vi "LoadShotSetting.vi"(10 "Shot Number":i32, 11 "Experiment State in":T17={"error"={"status"=FALSE, "code"=0, "source"=""}, "Digitizer DAQmx Tasks"={"TaskArray"=[]}, "DAQ Settings"={"Channel Settings"=[], "Card Settings"=[]}, "Synchronization Settings"={"Synchronizer 0"="", "source terminal"="", "Synchronizer 1"="PXI1Slot2"}, "DAQ Data"=[], "Next Shot#"="", "System Message"="", "User Shot Notes"="", "Timing Settings"={"Timing Card Settings"=[], "Timing Channel Settings"=[]}, "Timing Tasks"={"TaskArray"=[]}, "Tree"="", "Time Card/Channels"=[], "DAQ Card/Channels"=[], "Program Version"="", "RIO Settings"={"Channel Settings"=[], "Card Settings"=[]}, "RIO References"={"Reference Array"=[]}, "RIO Data"={"RIO Deleaved Data"=[], "Raw Readout"=[]}, "RIO Card/Channels"=[3, 8], "DIO Channels"=0, "DIO Settings"={"DIO Channel Array"=[]}, "Global Settings"={"Initial Background Values"={"Reference Shot #"=0.0, "Background pressure [Torr]"=0.0, "Cryo temp [V]"=0.0, "Cryo temp [K]"=0.0, "Cryotemp Calibration File"=path ""}, "Gas Puffing"={"Gas A type"="N", "Gas B type"="N", "Gas C type"="N", "Gas A pressure [psi]"=0.0, "Gas B pressure [psi]"=0.0, "Gas C pressure [psi]"=0.0, "Innner Electrode"="", "Middle Electrode"="", "Outer Electrode"="", "Gas A bottle pressure [psi]"=0.0, "Gas B bottle pressure [psi]"=0.0, "Gas C bottle pressure [psi]"=0.0}, "PSU Voltages"={"Bias1 Voltage [V]"=0.0, "Bias2 Voltage [V]"=0.0, "PSU1 Voltage [V]"=0.0, "Puff-PSU1 CH1 Voltage [V]"=0.0, "Puff-PSU1 CH2 Voltage [V]"=0.0, "Puff-PSU1 CH3 Voltage [V]"=0.0, "PSU2 Voltage [V]"=0.0, "PSU3 Voltage [V]"=0.0}, "TEK 2024B Details"={"CH1"="", "CH2"="", "CH3"="", "CH4"="", "CH1 Ground State"="Grounded", "CH2 Ground State"="Grounded", "CH3 Ground State"="Grounded", "CH4 Ground State"="Grounded"}}, "Calibrations"={"CryoTemp"={"Comment"="", "X"=[], "Y"=[]}, "PSU2 Tach"={"Comment"="", "X"=[], "Y"=[]}, "PSU3 Tach"={"Comment"="", "X"=[], "Y"=[]}, "PSU2 RevTach"={"Comment"="", "X"=[], "Y"=[]}, "PSU3 RevTach"={"Comment"="", "X"=[], "Y"=[]}}, "Tach Tasks"={"PSU2 task"="", "PSU3 task"=""}, "PSU2 Panel Settings"={"PSU2 DIO channels"={"Charge relay DIO"="DAQ0/port0/line3", "Dump relay DIO"="DAQ0/port0/line4", "HV Arm DIO"="DAQ0/port0/line5", "HV On DIO"="DAQ0/port0/line6"}, "PSU2 Tachometer Controls"={"PSU2 Tach Calibration"=path "Z:/Data/Calibration/Tachometer", "PSU2 Charging Voltage [kV]"=0.0, "PSU2 Tach Counter"="DAQ0/port0/line3"}, "PSU2 Reverse Tachometer Controls"={"PSU2 RevTach Calibration"=path "Z:/Data/Calibration/Reverse Tachometer/PSU2_RevTachCalibration.csv", "PSU2 bank Voltage [kV]"=0.0, "PSU2 RevTach Counter"=""}}, "PSU3 Panel Settings"={"PSU3 DIO channels"={"Charge relay DIO"="DAQ0/port0/line5", "Dump relay DIO"="DAQ0/port0/line6", "HV Arm DIO"="", "HV On DIO"="DAQ0/port0/line6"}, "PSU3 Tachometer Controls"={"PSU3 Tach Calibration"=path "Z:/Data/Calibration/Reverse Tachometer/PSU3_RevTachCalibration.csv", "PSU3 Charging Voltage [kV]"=0.0, "PSU3 Tach Counter"=""}, "PSU3 Reverse Tachometer Controls"={"PSU3 RevTach Calibration"=path "Z:/Data/Calibration/Reverse Tachometer/PSU3_RevTachCalibration.csv", "PSU3 bank Voltage [kV]"=0.0, "PSU3 RevTach Counter"=""}}} {"Global Settings"."Initial Background Values"."Cryo temp [K]" format="%#_4g"; "RIO Settings"."Card Settings"."Digital High \nPass Filter k" items=["10"=21, "9"=19, "8"=17, "7"=15, "6"=13, "5"=11, "4"=9, "3"=7, "2"=5, "Off"=0]; "RIO Settings"."Card Settings"."Sample Rate" format="%#_3p"; "Timing Settings"."Timing Channel Settings"."FrontPanelTime" format="%.3p"; "Timing Settings"."Timing Channel Settings"."Pulse width (s)" format="%.3p"; "Timing Settings"."Timing Channel Settings"."Delay (s)" format="%.3p"; "DAQ Settings"."Card Settings"."Global Edge Type" items=["Rising"=10280, "Falling"=10171]; "DAQ Settings"."Card Settings"."Sample Rate" format="%#_3p"}) -> (0 "Initialized RIO Array":T10 {"Card Settings"."Digital High \nPass Filter k" items=["10"=21, "9"=19, "8"=17, "7"=15, "6"=13, "5"=11, "4"=9, "3"=7, "2"=5, "Off"=0]; "Card Settings"."Start Time" format="%#_3p"; "Card Settings"."End Time" format="%#_3p"; "Card Settings"."Rate" format="%#_3p"}, 1 "Initialized DAQ Array":T48(array[cluster]) {"Card Settings"."Start Time" format="%#_3p"; "Card Settings"."End Time" format="%#_3p"; "Card Settings"."Rate" format="%#_3p"}, 2 "Initialized Timing Array":T43[](array[typedef]) {"Timing Sequence"."Pulse Width [s]" format="%#.2p"; "Timing Sequence"."Dt" format="%.2p"; "Timing Sequence"."Time" format="%.2p"}, 3 "Experiment State OUT":T17={"error"={"status"=FALSE, "code"=0, "source"=""}, "Digitizer DAQmx Tasks"={"TaskArray"=[]}, "DAQ Settings"={"Channel Settings"=[], "Card Settings"=[]}, "Synchronization Settings"={"Synchronizer 0"="", "source terminal"="", "Synchronizer 1"="PXI1Slot2"}, "DAQ Data"=[], "Next Shot#"="", "System Message"="", "User Shot Notes"="", "Timing Settings"={"Timing Card Settings"=[], "Timing Channel Settings"=[]}, "Timing Tasks"={"TaskArray"=[]}, "Tree"="", "Time Card/Channels"=[], "DAQ Card/Channels"=[], "Program Version"="", "RIO Settings"={"Channel Settings"=[], "Card Settings"=[]}, "RIO References"={"Reference Array"=[]}, "RIO Data"={"RIO Deleaved Data"=[], "Raw Readout"=[]}, "RIO Card/Channels"=[3, 8], "DIO Channels"=0, "DIO Settings"={"DIO Channel Array"=[]}, "Global Settings"={"Initial Background Values"={"Reference Shot #"=0.0, "Background pressure [Torr]"=0.0, "Cryo temp [V]"=0.0, "Cryo temp [K]"=0.0, "Cryotemp Calibration File"=path ""}, "Gas Puffing"={"Gas A type"="N", "Gas B type"="N", "Gas C type"="N", "Gas A pressure [psi]"=0.0, "Gas B pressure [psi]"=0.0, "Gas C pressure [psi]"=0.0, "Innner Electrode"="", "Middle Electrode"="", "Outer Electrode"="", "Gas A bottle pressure [psi]"=0.0, "Gas B bottle pressure [psi]"=0.0, "Gas C bottle pressure [psi]"=0.0}, "PSU Voltages"={"Bias1 Voltage [V]"=0.0, "Bias2 Voltage [V]"=0.0, "PSU1 Voltage [V]"=0.0, "Puff-PSU1 CH1 Voltage [V]"=0.0, "Puff-PSU1 CH2 Voltage [V]"=0.0, "Puff-PSU1 CH3 Voltage [V]"=0.0, "PSU2 Voltage [V]"=0.0, "PSU3 Voltage [V]"=0.0}, "TEK 2024B Details"={"CH1"="", "CH2"="", "CH3"="", "CH4"="", "CH1 Ground State"="Grounded", "CH2 Ground State"="Grounded", "CH3 Ground State"="Grounded", "CH4 Ground State"="Grounded"}}, "Calibrations"={"CryoTemp"={"Comment"="", "X"=[], "Y"=[]}, "PSU2 Tach"={"Comment"="", "X"=[], "Y"=[]}, "PSU3 Tach"={"Comment"="", "X"=[], "Y"=[]}, "PSU2 RevTach"={"Comment"="", "X"=[], "Y"=[]}, "PSU3 RevTach"={"Comment"="", "X"=[], "Y"=[]}}, "Tach Tasks"={"PSU2 task"="", "PSU3 task"=""}, "PSU2 Panel Settings"={"PSU2 DIO channels"={"Charge relay DIO"="DAQ0/port0/line3", "Dump relay DIO"="DAQ0/port0/line4", "HV Arm DIO"="DAQ0/port0/line5", "HV On DIO"="DAQ0/port0/line6"}, "PSU2 Tachometer Controls"={"PSU2 Tach Calibration"=path "Z:/Data/Calibration/Tachometer", "PSU2 Charging Voltage [kV]"=0.0, "PSU2 Tach Counter"="DAQ0/port0/line3"}, "PSU2 Reverse Tachometer Controls"={"PSU2 RevTach Calibration"=path "Z:/Data/Calibration/Reverse Tachometer/PSU2_RevTachCalibration.csv", "PSU2 bank Voltage [kV]"=0.0, "PSU2 RevTach Counter"=""}}, "PSU3 Panel Settings"={"PSU3 DIO channels"={"Charge relay DIO"="DAQ0/port0/line5", "Dump relay DIO"="DAQ0/port0/line6", "HV Arm DIO"="", "HV On DIO"="DAQ0/port0/line6"}, "PSU3 Tachometer Controls"={"PSU3 Tach Calibration"=path "Z:/Data/Calibration/Reverse Tachometer/PSU3_RevTachCalibration.csv", "PSU3 Charging Voltage [kV]"=0.0, "PSU3 Tach Counter"=""}, "PSU3 Reverse Tachometer Controls"={"PSU3 RevTach Calibration"=path "Z:/Data/Calibration/Reverse Tachometer/PSU3_RevTachCalibration.csv", "PSU3 bank Voltage [kV]"=0.0, "PSU3 RevTach Counter"=""}}} {"Global Settings"."Initial Background Values"."Cryo temp [K]" format="%#_4g"; "RIO Settings"."Card Settings"."Digital High \nPass Filter k" items=["10"=21, "9"=19, "8"=17, "7"=15, "6"=13, "5"=11, "4"=9, "3"=7, "2"=5, "Off"=0]; "RIO Settings"."Card Settings"."Sample Rate" format="%#_3p"; "Timing Settings"."Timing Channel Settings"."FrontPanelTime" format="%.3p"; "Timing Settings"."Timing Channel Settings"."Pulse width (s)" format="%.3p"; "Timing Settings"."Timing Channel Settings"."Delay (s)" format="%.3p"; "DAQ Settings"."Card Settings"."Global Edge Type" items=["Rising"=10280, "Falling"=10171]; "DAQ Settings"."Card Settings"."Sample Rate" format="%#_3p"}, 4 "Initialized DIO Cluster":T7, 5 "PSU3 Control Panel":T1={"HV Off State"=FALSE, "HV On State"=FALSE, "HV Arm"=FALSE, "HV On"=FALSE, "Charge relay DIO"="DAQ0/port0/line3", "Dump relay DIO"="DAQ0/port0/line4", "HV Arm DIO"="DAQ0/port0/line5", "HV On DIO"="DAQ0/port0/line6", "Bank Voltage [kV]"={0.0, 0.0}, "Vdemand Counter"="Timing1/ctr1", "RevTach Calibration"=path "Z:/Data/Calibration/Reverse Tachometer/PSU2_RevTachCalibration.csv", "Vdemand"=FALSE, "Vmeasure Counter"="Timing1/ctr2", "Tach Calibration"=path "Z:/Data/Calibration/Tachometer/PSU2_TachCalibration.csv", "Vmeasure"=FALSE, "Vdemand [kV]"=0.0, "Charge Relay"=FALSE, "Dump Relay"=FALSE} {"Bank Voltage [kV]" scale=0.01..10.0 scale format="%#_3g"}, 6 "Global Settings":T2={"Initial Background Values"={"Reference Shot #"=0.0, "Background pressure [Torr]"=0.0, "Cryo temp [V]"=0.0, "Cryo temp [K]"=0.0, "Cryotemp Calibration File"=path ""}, "Gas Puffing"={"Gas A type"="N", "Gas B type"="N", "Gas C type"="N", "Gas A pressure [psi]"=0.0, "Gas B pressure [psi]"=0.0, "Gas C pressure [psi]"=0.0, "Innner Electrode"="", "Middle Electrode"="", "Outer Electrode"="", "Gas A bottle pressure [psi]"=0.0, "Gas B bottle pressure [psi]"=0.0, "Gas C bottle pressure [psi]"=0.0}, "PSU Voltages"={"Bias1 Voltage [V]"=0.0, "Bias2 Voltage [V]"=0.0, "PSU1 Voltage [V]"=0.0, "Puff-PSU1 CH1 Voltage [V]"=0.0, "Puff-PSU1 CH2 Voltage [V]"=0.0, "Puff-PSU1 CH3 Voltage [V]"=0.0, "PSU2 Voltage [V]"=0.0, "PSU3 Voltage [V]"=0.0}, "TEK 2024B Details"={"CH1"="", "CH2"="", "CH3"="", "CH4"="", "CH1 Ground State"="Grounded", "CH2 Ground State"="Grounded", "CH3 Ground State"="Grounded", "CH4 Ground State"="Grounded"}} {"Initial Background Values"."Cryo temp [K]" format="%#_4g"}, 7 "PSU2 Control Panel":T1={"HV Off State"=FALSE, "HV On State"=FALSE, "HV Arm"=FALSE, "HV On"=FALSE, "Charge relay DIO"="DAQ0/port0/line3", "Dump relay DIO"="DAQ0/port0/line4", "HV Arm DIO"="DAQ0/port0/line5", "HV On DIO"="DAQ0/port0/line6", "Bank Voltage [kV]"={0.0, 0.0}, "Vdemand Counter"="Timing1/ctr1", "RevTach Calibration"=path "Z:/Data/Calibration/Reverse Tachometer/PSU2_RevTachCalibration.csv", "Vdemand"=FALSE, "Vmeasure Counter"="Timing1/ctr2", "Tach Calibration"=path "Z:/Data/Calibration/Tachometer/PSU2_TachCalibration.csv", "Vmeasure"=FALSE, "Vdemand [kV]"=0.0, "Charge Relay"=FALSE, "Dump Relay"=FALSE} {"Bank Voltage [kV]" scale=0.01..10.0 scale format="%#_3g"}, 8 "Shot Notes":string)   [LabVIEW 2015]
uses:
  Controls/DAQ Card Channel Array.ctl
  Controls/DAQ Channel Settings.ctl
  Controls/DAQ Card Settings.ctl
  Controls/TimingControl.ctl
  Controls/TimingControlChannel.ctl
  Controls/ExperimentStateCluster.ctl
  Controls/DigitizerSettingsChannelSettings.ctl
  Controls/DigitizerSettingsCardSettingsArray.ctl
  Controls/DigitizerSettingsCardSettings.ctl
  Controls/TimingSettings.ctl
  Controls/TimingCardSettings.ctl
  Controls/TimingChannelSettings.ctl
  Controls/RIOSettingsExperimentStateCluster.ctl
  Controls/RIOChannelSettingsArrayExperimentStateCluster.ctl
  Controls/RIOSettingsChannelSettings.ctl
  Controls/RIOSettingsCardSettingsArray.ctl
  Controls/RIOSettingsCardSettings.ctl
  <vilib>/userdefined/High Color/nirio_resource_hc.ctl
  Controls/DigitalHighPassFilter.ctl
  Controls/RIOData.ctl
  Controls/DIOChannel.ctl
  Controls/Global Settings/GlobalSettings.ctl
  Controls/Global Settings/InitialBackgroundValues.ctl
  Controls/Global Settings/GasPuffing.ctl
  Controls/Global Settings/PSUVoltages.ctl
  Controls/Global Settings/ScopeDetails.ctl
  Controls/Calibrations/Calibrations.ctl
  Controls/Calibrations/CryoTemoCalibration.ctl
  Controls/Calibrations/PSU2TachCalibration.ctl
  Controls/Calibrations/PSU3TachCalibration.ctl
  Controls/TachTasks.ctl
  Controls/PSU2PanelSettings.ctl
  Controls/PSU2DIOChannels.ctl
  Controls/PSU2TachometerControls.ctl
  Controls/PSU2ReverseTachometerControls.ctl
  Controls/PSU3PanelSettings.ctl
  Controls/PSU3DIOChannels.ctl
  Controls/PSU3TachometerControls.ctl
  Controls/PSU3ReverseTachometerControls.ctl
  Controls/RIOCardArray.ctl
  Controls/RIOCardElement.ctl
  Controls/RIOCardChannelArray.ctl
  Controls/RIOChannelSettings.ctl
  Controls/RIOCardSettings.ctl
  Controls/DIOTypedef.ctl
  Controls/DIOChannelArray.ctl
  Controls/PSUPanel-Arming.ctl
panel:
  # "On/Off      Channel                     Name"
  # "Channel                                                  Name                         Atten [dB]            Card Settings"
  # "Sampling Rate [1/s]"
  # "Start Time [s]"
  # "End Time [s]"
  # "Sampling Rate [1/s]"
  # "Start Time [s]"
  # "End Time [s]"
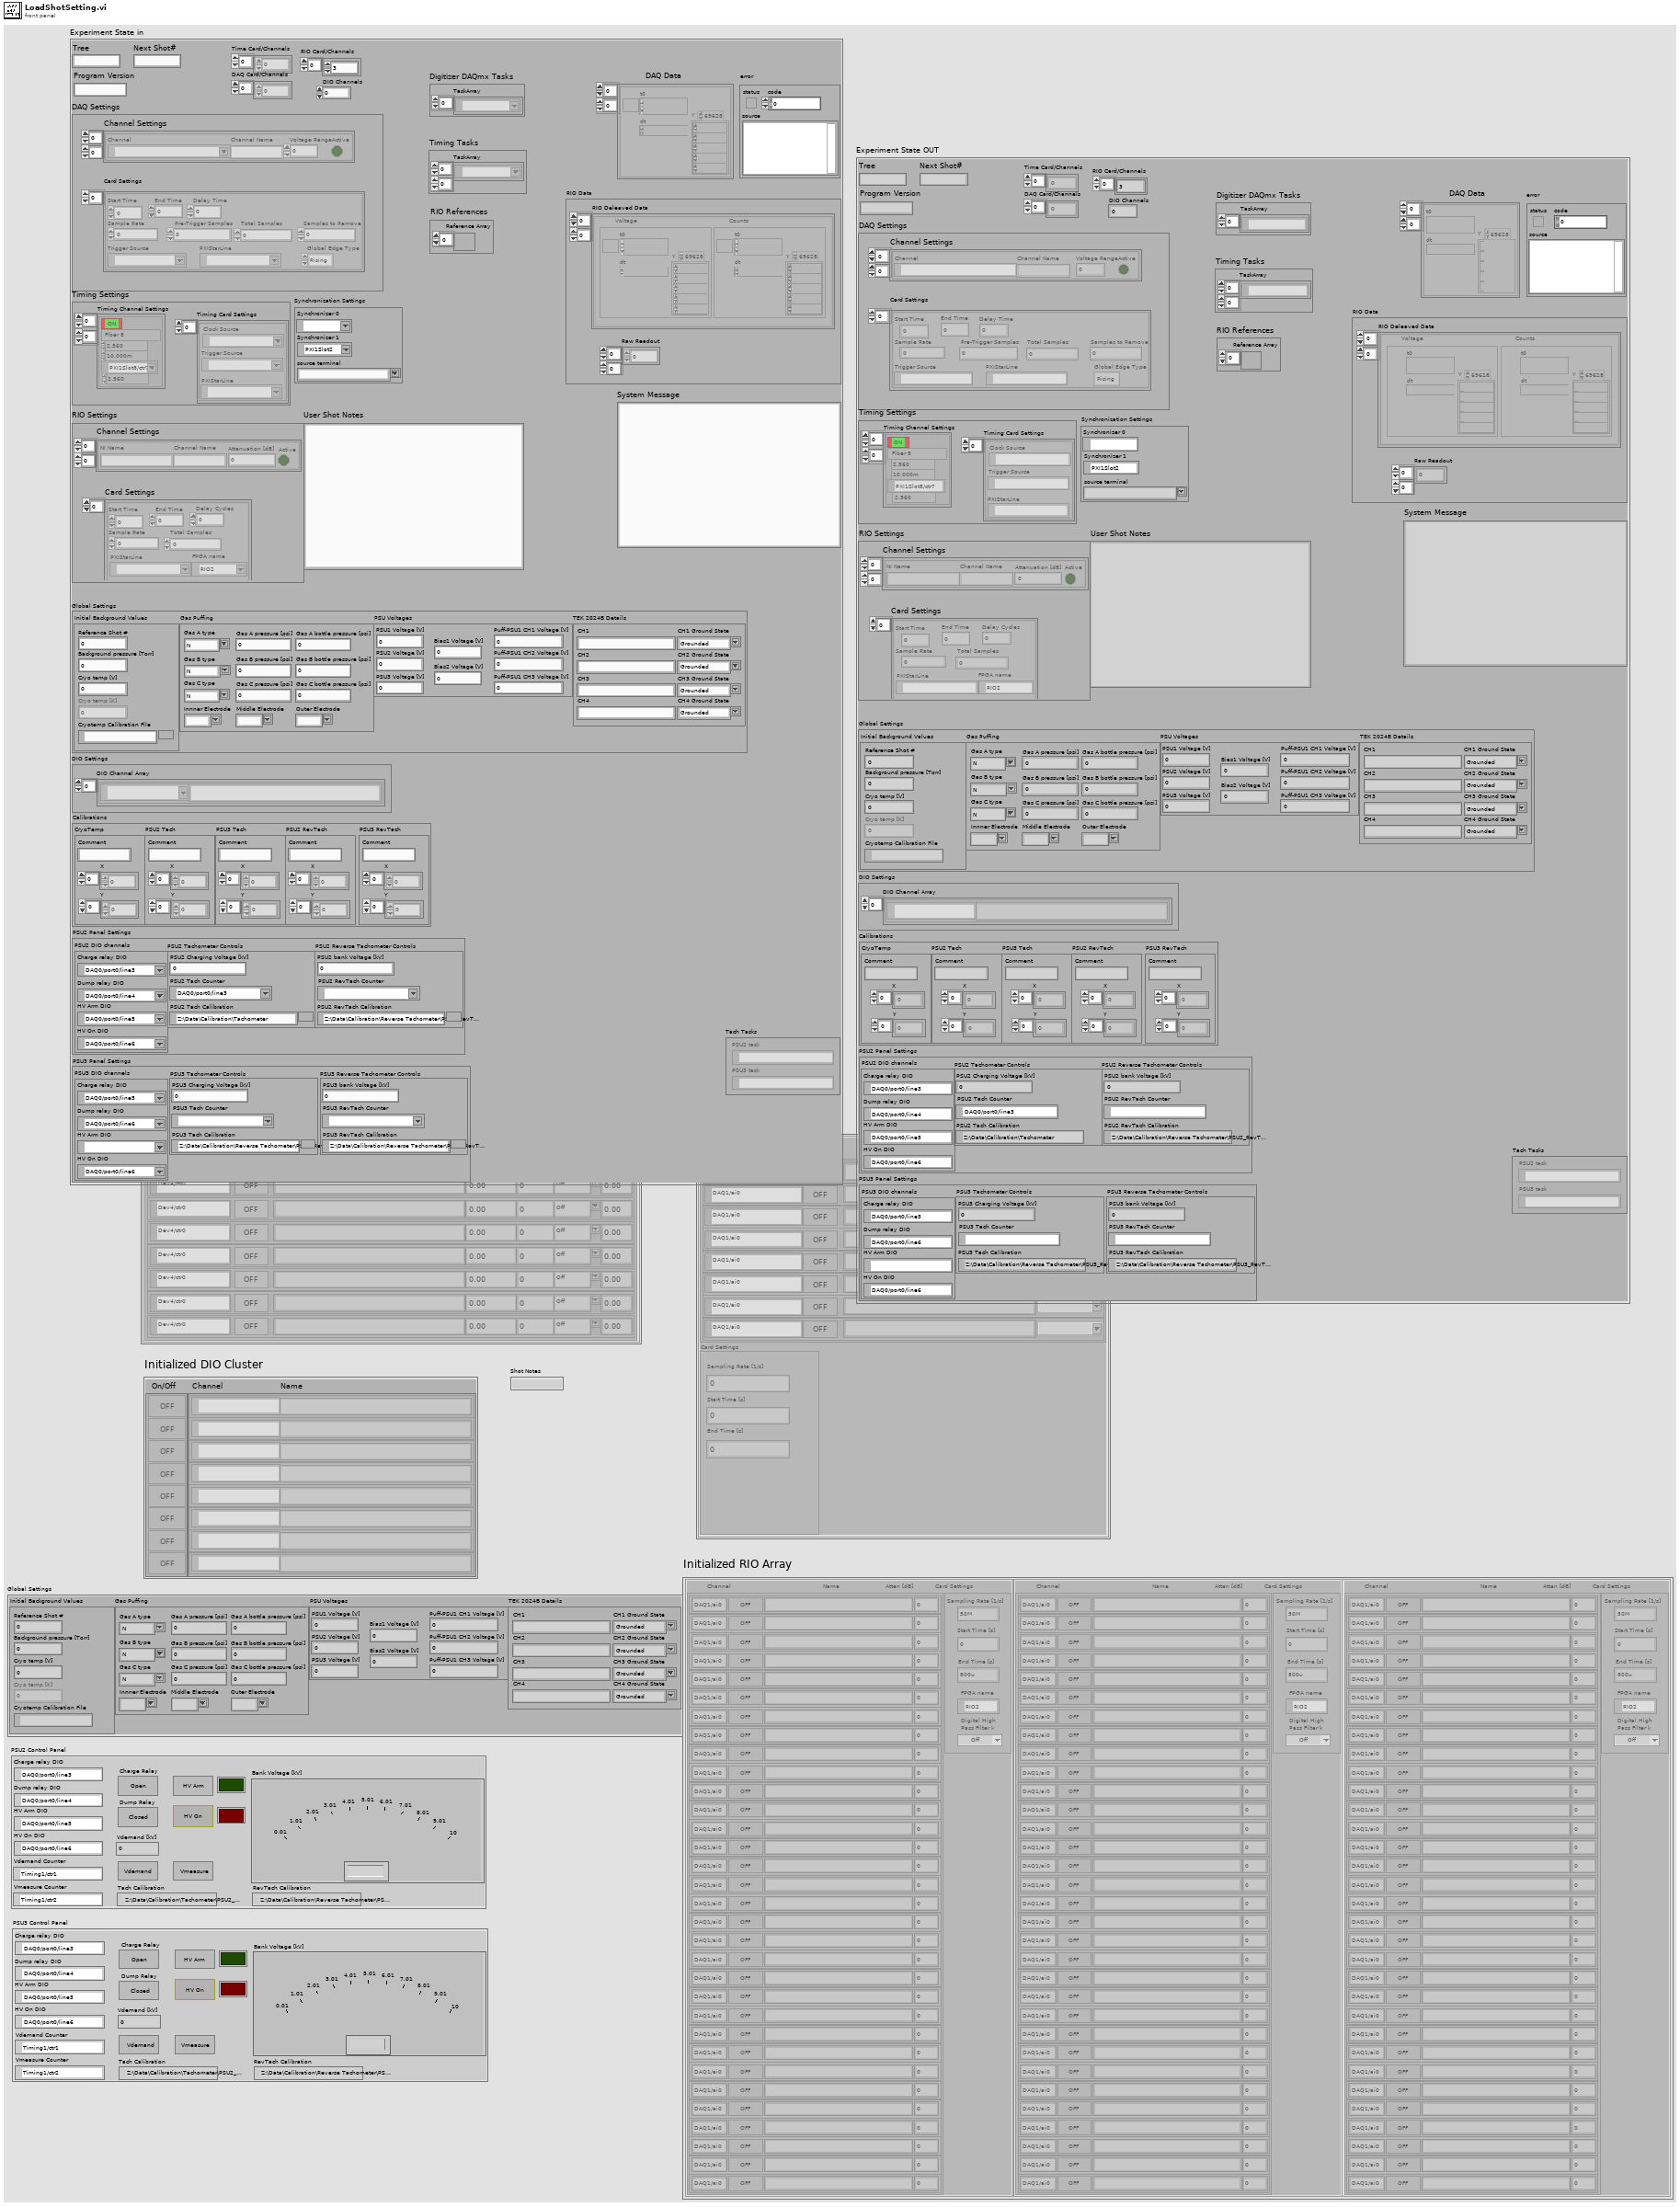
[diagram p1: front panel]
types:
  T1 = typedef "PSUPanel-Arming.ctl" = cluster{"HV Off State":bool, "HV On State":bool, "HV Arm":bool, "HV On":bool, "Charge relay DIO":tag, "Dump relay DIO":tag, "HV Arm DIO":tag, "HV On DIO":tag, "Bank Voltage [kV]":cluster{dbl, dbl}, "Vdemand Counter":tag, "RevTach Calibration":path, "Vdemand":bool, "Vmeasure Counter":tag, "Tach Calibration":path, "Vmeasure":bool, "Vdemand [kV]":dbl, "Charge Relay":bool, "Dump Relay":bool}
  T2 = typedef "GlobalSettings.ctl" = cluster{"Initial Background Values":T3, "Gas Puffing":T4, "PSU Voltages":T5, "TEK 2024B Details":T6}
  T3 = typedef "InitialBackgroundValues.ctl" = cluster{"Reference Shot #":dbl, "Background pressure [Torr]":dbl, "Cryo temp [V]":dbl, "Cryo temp [K]":dbl, "Cryotemp Calibration File":path}
  T4 = typedef "GasPuffing.ctl" = cluster{"Gas A type":string, "Gas B type":string, "Gas C type":string, "Gas A pressure [psi]":dbl, "Gas B pressure [psi]":dbl, "Gas C pressure [psi]":dbl, "Innner Electrode":string, "Middle Electrode":string, "Outer Electrode":string, "Gas A bottle pressure [psi]":dbl, "Gas B bottle pressure [psi]":dbl, "Gas C bottle pressure [psi]":dbl}
  T5 = typedef "PSUVoltages.ctl" = cluster{"Bias1 Voltage [V]":dbl, "Bias2 Voltage [V]":dbl, "PSU1 Voltage [V]":dbl, "Puff-PSU1 CH1 Voltage [V]":dbl, "Puff-PSU1 CH2 Voltage [V]":dbl, "Puff-PSU1 CH3 Voltage [V]":dbl, "PSU2 Voltage [V]":dbl, "PSU3 Voltage [V]":dbl}
  T6 = typedef "ScopeDetails.ctl" = cluster{"CH1":string, "CH2":string, "CH3":string, "CH4":string, "CH1 Ground State":string, "CH2 Ground State":string, "CH3 Ground State":string, "CH4 Ground State":string}
  T7 = typedef "DIOTypedef.ctl" = cluster{"DIO Booleans":bool[], "DIO Channel Array":T8}
  T8 = typedef "DIOChannelArray.ctl" = T9[]
  T9 = typedef "DIOChannel.ctl" = cluster{"Channel Name":string, "NI Name":tag}
  T10 = typedef "RIOCardArray.ctl" = T11[][]
  T11 = typedef "RIOCardElement.ctl" = cluster{"RIO Channel Array":T12, "Card Settings":T14}
  T12 = typedef "RIOCardChannelArray.ctl" = T13[]
  T13 = typedef "RIOChannelSettings.ctl" = cluster{"Active":bool, "Channel Name":string, "NI Name":string, "Attenutaion [dB]":i32}
  T14 = typedef "RIOCardSettings.ctl" = cluster{"Rate":dbl, "End Time":dbl, "Start Time":dbl, "FPGA name":T15, "Digital High \nPass Filter k":T16}
  T15 = typedef "nirio_resource_hc.ctl" = tag
  T16 = typedef "DigitalHighPassFilter.ctl" = u16
  T17 = typedef "ExperimentStateCluster.ctl" = cluster{"error":errorcluster, "Digitizer DAQmx Tasks":cluster{"TaskArray":refnum<k21>[]}, "DAQ Settings":cluster{"Channel Settings":T18[][], "Card Settings":T19}, "Synchronization Settings":cluster{"Synchronizer 0":refnum<k15>, "source terminal":string, "Synchronizer 1":refnum<k15>}, "DAQ Data":waveform(dbl)[][], "Next Shot#":string, "System Message":string, "User Shot Notes":string, "Timing Settings":T21, "Timing Tasks":cluster{"TaskArray":refnum<k21>[][]}, "Tree":string, "Time Card/Channels":i32[], "DAQ Card/Channels":i32[], "Program Version":string, "RIO Settings":T24, "RIO References":cluster{"Reference Array":refnum<k20>[]}, "RIO Data":T29, "RIO Card/Channels":i32[], "DIO Channels":i32, "DIO Settings":cluster{"DIO Channel Array":T9[]}, "Global Settings":T2, "Calibrations":T30, "Tach Tasks":T34, "PSU2 Panel Settings":T35, "PSU3 Panel Settings":T39}
  T18 = typedef "DigitizerSettingsChannelSettings.ctl" = cluster{"Channel":tag, "Channel Name":string, "Voltage Range":dbl, "Active":bool}
  T19 = typedef "DigitizerSettingsCardSettingsArray.ctl" = T20[]
  T20 = typedef "DigitizerSettingsCardSettings.ctl" = cluster{"Start Time":dbl, "End Time":dbl, "Sample Rate":dbl, " Pre-Trigger Samples":u32, "Total Samples":i32, "Samples to Remove":u32, "Trigger Source":tag, "Global Edge Type":i32, "PXIStarLine":tag, "Delay Time":dbl}
  T21 = typedef "TimingSettings.ctl" = cluster{"Timing Card Settings":T22[], "Timing Channel Settings":T23[][]}
  T22 = typedef "TimingCardSettings.ctl" = cluster{"Trigger Source":tag, "Clock Source":tag, "PXIStarLine":tag}
  T23 = typedef "TimingChannelSettings.ctl" = cluster{"Delay (s)":dbl, "Pulse width (s)":dbl, "Active":bool, "Channel Name":string, "counter":tag, "FrontPanelTime":dbl}
  T24 = typedef "RIOSettingsExperimentStateCluster.ctl" = cluster{"Channel Settings":T25, "Card Settings":T27}
  T25 = typedef "RIOChannelSettingsArrayExperimentStateCluster.ctl" = T26[][]
  T26 = typedef "RIOSettingsChannelSettings.ctl" = cluster{"Channel Name":string, "Active":bool, "NI Name":string, "Attenuation [dB]":i32}
  T27 = typedef "RIOSettingsCardSettingsArray.ctl" = T28[]
  T28 = typedef "RIOSettingsCardSettings.ctl" = cluster{"Start Time":dbl, "End Time":dbl, "Sample Rate":dbl, "Total Samples":u64, "PXIStarLine":tag, "Delay Cycles":u64, "FPGA name":T15, "Digital High \nPass Filter k":T16}
  T29 = typedef "RIOData.ctl" = cluster{"RIO Deleaved Data":cluster{"Voltage":waveform(dbl), "Counts":waveform(i16)}[][], "Raw Readout":u64[][]}
  T30 = typedef "Calibrations.ctl" = cluster{"CryoTemp":T31, "PSU2 Tach":T32, "PSU3 Tach":T33, "PSU2 RevTach":T32, "PSU3 RevTach":T33}
  T31 = typedef "CryoTemoCalibration.ctl" = cluster{"Comment":string, "X":dbl[], "Y":dbl[]}
  T32 = typedef "PSU2TachCalibration.ctl" = cluster{"Comment":string, "X":dbl[], "Y":dbl[]}
  T33 = typedef "PSU3TachCalibration.ctl" = cluster{"Comment":string, "X":dbl[], "Y":dbl[]}
  T34 = typedef "TachTasks.ctl" = cluster{"PSU2 task":refnum<k21>, "PSU3 task":refnum<k21>}
  T35 = typedef "PSU2PanelSettings.ctl" = cluster{"PSU2 DIO channels":T36, "PSU2 Tachometer Controls":T37, "PSU2 Reverse Tachometer Controls":T38}
  T36 = typedef "PSU2DIOChannels.ctl" = cluster{"Charge relay DIO":tag, "Dump relay DIO":tag, "HV Arm DIO":tag, "HV On DIO":tag}
  T37 = typedef "PSU2TachometerControls.ctl" = cluster{"PSU2 Tach Calibration":path, "PSU2 Charging Voltage [kV]":dbl, "PSU2 Tach Counter":tag}
  T38 = typedef "PSU2ReverseTachometerControls.ctl" = cluster{"PSU2 RevTach Calibration":path, "PSU2 bank Voltage [kV]":dbl, "PSU2 RevTach Counter":tag}
  T39 = typedef "PSU3PanelSettings.ctl" = cluster{"PSU3 DIO channels":T40, "PSU3 Tachometer Controls":T41, "PSU3 Reverse Tachometer Controls":T42}
  T40 = typedef "PSU3DIOChannels.ctl" = cluster{"Charge relay DIO":tag, "Dump relay DIO":tag, "HV Arm DIO":tag, "HV On DIO":tag}
  T41 = typedef "PSU3TachometerControls.ctl" = cluster{"PSU3 Tach Calibration":path, "PSU3 Charging Voltage [kV]":dbl, "PSU3 Tach Counter":tag}
  T42 = typedef "PSU3ReverseTachometerControls.ctl" = cluster{"PSU3 RevTach Calibration":path, "PSU3 bank Voltage [kV]":dbl, "PSU3 RevTach Counter":tag}
  T43 = typedef "TimingControl.ctl" = cluster{"Timing Sequence":T44[]}
  T44 = typedef "TimingControlChannel.ctl" = cluster{"Active":bool, "counter":tag, "Channel Name":string, "Time":dbl, "Increment":string, "Dt":dbl, "Pulse Width [s]":dbl}
  T45 = typedef "DAQ Card Channel Array.ctl" = T46[]
  T46 = typedef "DAQ Channel Settings.ctl" = cluster{"Active":bool, "Channel Name":string, "Channel":tag, "Voltage Range":string}
  T47 = typedef "DAQ Card Settings.ctl" = cluster{"Rate":dbl, "End Time":dbl, "Start Time":dbl}
  T48 = cluster{"DAQ Channel Array":T45, "Card Settings":T47}[]
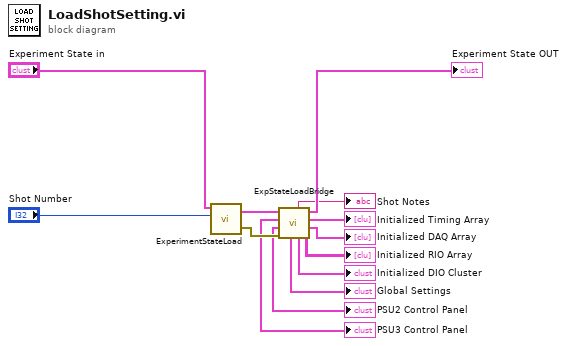
[diagram p0: block diagram]
diagram:
  n1 = call "ExperimentStateLoad.vi"("Previous Shot #"="Shot Number", "Current ExpState IN"="Experiment State in") -> ("Error out"=w11:errorcluster, "Updated ExpState OUT"=w12:T17)  [unwired: 2 in]
  n2 = call "ExpStateLoadBridge.vi"("Error In"=w11, "Experiment State IN"=w12) -> ("Load RIO Array"=→"Initialized RIO Array":T10, "Load DAQ Array"=→"Initialized DAQ Array":T48, "Load Timing Array"=→"Initialized Timing Array":T43[], "Experiment State OUT"=→"Experiment State OUT":T17, "Load DIO Cluster"=→"Initialized DIO Cluster":T7, "Shot Notes"=→"Shot Notes":string, "Global Settings"=→"Global Settings":T2, "PSU2 Control Panel"=→"PSU2 Control Panel":T1, "PSU3 Control Panel"=→"PSU3 Control Panel":T1)  [unwired: 1 in]
